vi "TestService.vi"   [LabVIEW 2011]
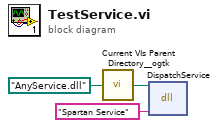
[diagram p0: block diagram]
diagram:
  n1 = call <userlib>:"Current VIs Parent Directory__ogtk.vi"("Relative path (.)"=path "AnyService.dll") -> ("Parent Directory (+ Relative)"=w1:path)  [unwired: 4 out]
  n2 = dll-call lib="C:/DEVELOPMENT/SPARTAN/server/service/AnyService.dll" fn="DispatchService"(path in=w1, "serviceName"="Spartan Service") -> ()  [unwired: 2 in, 4 out]
